vi "Server_REPL_Read.vi"(8 "error in (no error)":errorcluster, 9 "Clear":bool, 11 "Server":path) -> (0 "error out":errorcluster, 1 "Running?":bool, 2 "REPL":string)   [LabVIEW 2020]
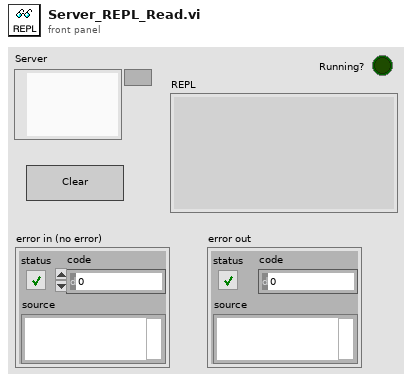
[diagram p1: front panel]
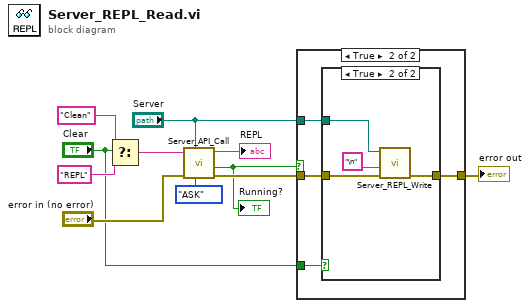
[diagram p0: block diagram]
diagram:
  n1 = Select(t="Clean" ("url"), s="Clear", f="REPL" ("url")) -> (s? t:f=w8:string)
  n2 = call "Server_API_Call.vi"("Server"="Server", "Direction"=enum16{"ASK", "TELL"}."ASK", "error in (no error)"="error in (no error)", "cmd"=w8) -> ("error out"=w3:errorcluster, "Running?"=w1:bool, "Read from Server"=→"REPL":string)  [unwired: 5 in]
  "Running?" <- w1
  n3 = case shown="True" w1 {
    tunnel: "Clear" -> [_ w16]
    tunnel: [w12 w15] -> w6
    tunnel: w3 -> [w12 w14]
    tunnel: "Server" -> [_ w13]
    frame False {
    }
    frame True {
      n4 = case shown="True" w16 {
        tunnel: w14 -> [w17 w21]
        tunnel: [w17 w20] -> w15
        tunnel: w13 -> [_ w19]
        frame False {
        }
        frame True {
          n5 = call "Server_REPL_Write.vi"("error in (no error)"=w21, "Code"="\n", "Server"=w19) -> ("error out"=w20:errorcluster)  [unwired: 8 in]
        }
      }
    }
  }
  "error out" <- w6
